vi "Start Traverse System.vi"(8 "error in":errorcluster, 10 "VISA resource name":refnum<visa-resource-name>, 11 "Water Tunnel Results in":refnum<class "Water Tunnel Results.lvclass">) -> (0 "error out":errorcluster, 3 "Water Tunnel Results out":refnum<class "Water Tunnel Results.lvclass">)   [LabVIEW 2019, in "Results.lvlib" / "Water Tunnel Results.lvclass"]
uses:
  Water Tunnel Results.lvclass
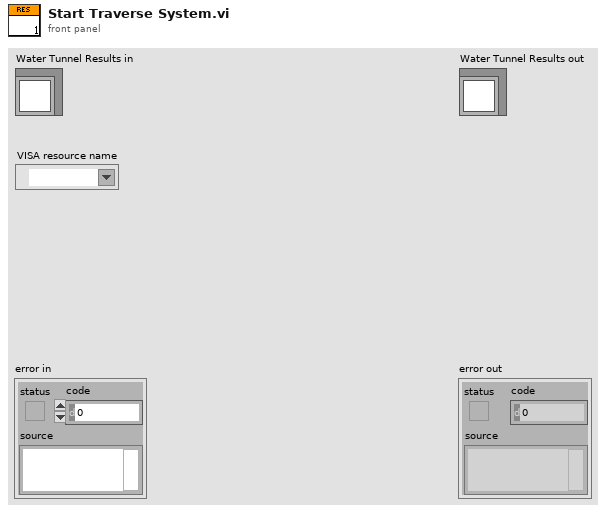
[diagram p1: front panel]
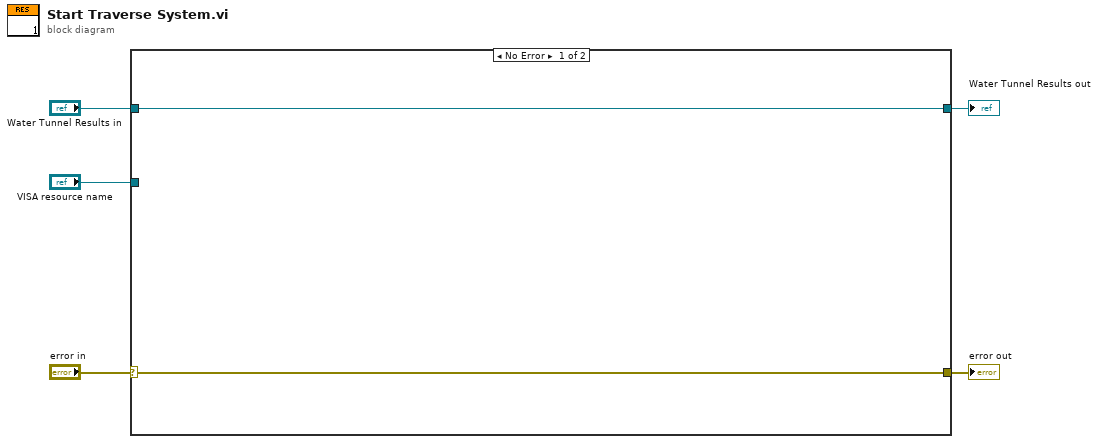
[diagram p0: block diagram]
diagram:
  n1 = case shown="No Error" "error in" {
    selector: "error in" -> [w6 w9]
    tunnel: [w6 w9] -> w4
    tunnel: [w7 w8] -> w2
    tunnel: "Water Tunnel Results in" -> [w7 w8]
    tunnel: "VISA resource name" -> [_ _]
    frame No Error {
    }
    frame Error {
    }
  }
  "error out" <- w4
  "Water Tunnel Results out" <- w2
